vi "Alle Frontpanels auslesen_IB.vi"(8 "error in (no error)":errorcluster caption="Fehler (Eingang, kein Fehler)") -> (0 "Fehler (Ausgang)":errorcluster)   [LabVIEW 2020, in "Sprachverwaltung.lvlib"]
uses:
  Sprachverwaltung.lvlib
  FGV Aktion Tabelle zerlegen.ctl
  Seiten.ctl
  EPA 1065/HovaCAL Interference verification/VI Interference Konfig.vi
  EPA 1065/HovaCAL Interference verification/HovaCAL Interference verificaton.lvlib
panel:
  # "Durch ausführen des VI´s werden alle Frontpanels\ndie man vorher hinzufügt ausgelesen"
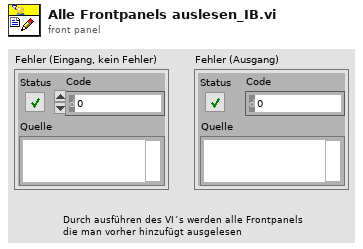
[diagram p1: front panel]
types:
  T1 = typedef "Sprachverwaltung.lvlib/Seiten.ctl" = enum16{"[ANLAGENGRENZWERTE]", "[LOG KONFIG]", "[GASZUORDNUNG]", "[ANLAGENÜBERSICHT]", "[GRAFIK]", "[CONFIG DIAGRAMME]", "[KONFIGURATION FTIR]", "[GASLISTE VERGLEICHEN]", "[ALGEBRAIC KONFIG]", "[FTIR DIAGNOSE]", "[ERWEITERTE KONFIG]", "[KONFIG AK]", "[STATUS STEUERUNG]", "[PID PARAMETER DRUCK-REGLER]", "[DICHTHEITSTEST]", "[T90 KONFIG]", "[T90]", "[HINTERGRUND]", "[SYSTEM EINSTELLUNGEN V2]", "[COPYRIGHT]", "[STATUSÜBERSICHT]", "[PASSWORTVERWALTUNG]", "[PASSWORT AENDERN]", "[FUNKTIONSTASTEN]", "[PNS]", "[DIAG PNS]", "[RUNTIME MENUE]", "[FAS06]", "[PERMANENT BEREICH]", "[RUNTIME BEENDEN]", "[SPEICHERN]", "[STOERMELDUNGEN]", "[STOERMELDEPUFFER]", "[STOERMELDE-KONFIG]", "[STOERMELDUNGSDATEI]", "[ERWEITERTE GASLISTE]", "[LINEARISIERUNG FTIR]", "[ARN TEST]", "[ARN PROTOKOLL]", "[FEHLER STEUERUNG]", "[POLYNOMKOEFFIZIENTEN]", "[KONFIG LINEARITY VERIFICATION]", "[AUTO LIN VERIFICATION]", "[GRAPHIK KURVEN]", "[EPA DICHTHEITSTEST]", "[REZEPT LADEN]", "[REZEPTWECHSEL]", "[DIAG ZYKLUSZEIT]", "[EPA KONTROLLE PARAMETER]", "[KONFIG GASTEILER]", "[KALIBRIERDATEN LADEN]", "[KONTROLLE PARAMETER VOR LIN]", "[KONFIGURATION KALIBRIERGASE]", "[INTERFERENCE VERIFICATION]", "[INTERFERENCE VERIFICATION 375]", "[INTERFERENCE PROTOKOLL 375]", "[INTERFERENCE PROTOKOLL]", "[INTERFERENCE HILFE]", "[SPUELEN]", "[GASTEILER SPUELEN]", "[GASTEILER KALIBRIEREN]", "[SENSOR KONFIGURATION]", "[KONFIGURATION PMA]", "[KALIBRIERDATEN]", "[KONFIGURATION FID]", "[ABB MANUELL KALIBRIEREN]", "[PMA MANUELL KALIBRIEREN]", "[SPRACHAUSWAHL]", "[SYS LOG HISTORY]", "[SYS LOG STATUS]", "[PNS UEBERSICHT]\t", "[CG TEST]", "[KONFIG CG CHECK]", "[HOVA MAIN]", "[HORIBA GDC]", "[BACKUP]", "[SPAN FAKTOREN]", "[CG POPUP]", "[AUTO CALIBRATION]", "[LIN V2]", "[O2 LEAKTEST]", "[CG TEST RESULT]", "[GASTEILER ABWEICHUNG]", "[EPA LIN CHECK PROTOKOLL]", "[LIN CHECK PROTOKOLL]", "[LEAK CHECK PROTOKOLL]", "[O2 LEAK PROTOKOLL]", "[HANG UP PROTOKOLL]", "[T90 PROTOKOLL]", "[SPRACHEDITOR]", "[SYSLOG CRIO MESSAGES]", "[SYSLOG PC MESSAGES]", "[SYSLOG PROPERTIES MESSAGES]", "[T90 EPA]", "[T90 EPA PDF]", "[SCHEDULER]", "[HINTERGRUND V2]", "[CG TEST PDF]", "[CHILLER EPA TEST]", "[CHILLER EPA PROTOKOLL]", "[FID O2 EPA TEST]", "[FID O2 EPA PROTOKOLL]", "[DRIFT EPA TEST]", "[DRIFT EPA PROTOKOLL]", "[PRE EPA TEST]", "[PRE EPA PROTOKOLL]", "[FID OPTIMIZATION]", "[FID OPTIMIZATION PDF]", "[FID RESPONSE FAKTOR]", "[KONFIG ZIRCONIA]", "[ZIRCONIA MANUELL KALIBRIEREN]", "[ARN EU PDF]", "[LEAK CHECK EU PDF]", "[T90 EU PDF]", "[LIN EU PDF]", "[NH3 DRIFT EU TEST]", "[NH3 DRIFT PDF]", "[NH3 INTERFERENCE PDF]", "[NH3 INTERFERENCE VERIFICATION]", "[CO2 INTERFERENCE VERIFICATION]", "[FILTER CHECK]", "[FILTER CHECK PDF]", "[CAN KONFIG]", "[GPS ANZEIGE]", "[BATTERY MANAGEMENT]", "[G-Shock]", "[AVL EFM]", "[Sensors EFM]", "[HovaCAL INTERFERENCE VERIFICATION]"}
  T2 = enum16{"Deutsch", "Englisch", "Französisch", "Italienisch"}
  T3 = typedef "Sprachverwaltung.lvlib/FGV Aktion Tabelle zerlegen.ctl" = enum16{"laden", "vereinzeln", "speichern"}
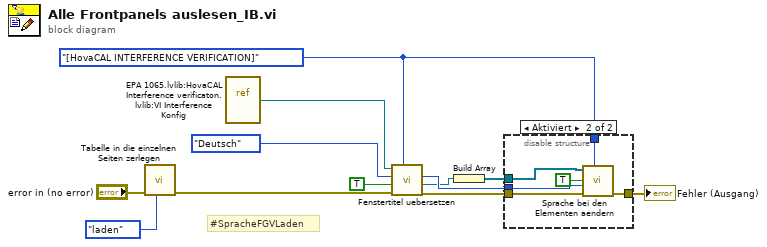
[diagram p0: block diagram]
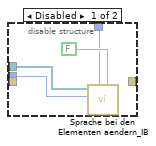
[diagram p2: hidden frame]
diagram:
  w2 = Seiten."[HovaCAL INTERFERENCE VERIFICATION]" ("Seiten")
  # "#SpracheFGVLaden"
  n1 = call "Tabelle in die einzelnen Seiten zerlegen.vi"("Aktion"=FGV_Aktion_Tabelle_zerlegen."laden", "error in (no error)"="error in (no error)") -> ("error out"=w7:errorcluster)  [unwired: 7 in, 2 out]
  n2 = vi-ref "EPA 1065.lvlib:HovaCAL Interference verificaton.lvlib:VI Interference Konfig.vi"() -> (w10:refnum<vi>)
  n3 = call "Fenstertitel uebersetzen.vi"("Index (Seite)"=w2, "error in (no error)"=w7, "Sprache verwenden"=TRUE, "Sprachauswahl"=T2."Deutsch", "Dieses VI"=w10) -> ("error out"=w4:errorcluster, "Dieses VI out"=w1:refnum<vi>, "Sprachauswahl out"=w3:u16)  [unwired: 3 in, 1 out]
  n4 = Build Array(w1) -> (w11:refnum<vi>[])
  n5 = disable-structure shown="Aktiviert" {
    disable-tunnel: w11 -> [w16 w22]
    disable-tunnel: w3 -> [w14 w21]
    disable-tunnel: [_ w19] -> w6
    disable-tunnel: w4 -> [_ w18]
    disable-tunnel: w2 -> [w13 w17]
    frame Disabled {
      n6 = call "Sprache bei den Elementen aendern_IB.vi"("Datei erstellen"=FALSE, "Index (Seite)"=w13, "Sprachauswahl"=w14, "VI Referenzen"=w16) -> ()  [unwired: 8 in]
    }
    frame Enabled {
      n7 = call "Sprache bei den Elementen aendern.vi"("Index"=w17, "Fehler (Eingang, kein Fehler)"=w18, "Sprachauswahl"=w21, "Index verwenden"=TRUE, "VI Referenzen"=w22) -> ("Fehler (Ausgang)"=w19:errorcluster)  [unwired: 5 in, 1 out]
    }
  }
  "Fehler (Ausgang)" <- w6
